vi "Avg_Example.vi"() -> ()   [LabVIEW 2019]
doc: "This example shows how to continously compute and show an averaged image.\nHere the camera class is operated in sequence mode and the required number of images also defines the number of images that will be averaged\nIt is a good starting point for writing own applications.\nBut it will not be fail save, i.e. doesnt react on errors, just handles them forward to the end\n\nUsage:\nSelect your required image count you want to average over before you start the program.\nOnce started, the camera class will be initialized and image record will start automatically.\nInside the acquisition loop the program will record the image sequence.\nThen it calculates the average image and shows it.\nBy using the ROI parameters you can crop the image to select certain regions\n\nBy clicking Quit Application the record will stop and will force an exit of the camera class"
uses:
  camera/Camera.lvclass
  <vilib>/picture/picture.llb/Draw 8-Bit Pixmap.vi
  <vilib>/picture/picture.llb/Draw True-Color Pixmap.vi
panel:
  out "colormap(U8)":u32[](array[numeric])
  out "Image(U16)":u16[][](graph)
  in  "Zoom [%]":i32(slide)=26 min=10 max=200 step=5 scale=10.0..200.0
  out "Image":picture
  out "rawImage":u16[][](array[numeric])
  in  "data_format":T1(ring)=enum."Mono16"
  out "Recorded Images":u32
  in  "Quit":bool
  in  "cropY1":u64=2 min=2 max=2048 step=1
  in  "cropX1":u64=2 min=2 max=2048 step=1
  in  "cropY0":u64=1 min=1 max=2047 step=1
  in  "cropX0":u64=1 min=1 max=2047 step=1
  out "Image Height":u64
  out "Image Width":u64
  in  "dwImgCount":u32=10 caption="Required Number of Images" max=4023
  out "Error":errorcluster {"code" format="%x"}
  # "This example shows how to continously compute and show an averaged image.\nHere the camera class is operated in sequence mode and the required number of images also defines the number of images that will be averaged\nIt is a good starting point for writing own applications.\nBut it will not be fail save, i.e. doesnt react on errors, just handles them forward to the end\n\nUsage:\nSelect your required image count you want to average over before you start the program.\nOnce started, the camera class will be initialized and image record will start automatically.\nInside the acquisition loop the program will record the image sequence.\nThen it calculates the average image and shows it.\nBy using the crop parameters you can crop the image to select certain regions\n\nBy clicking Quit Application the record will stop and will force an exit of the camera class"
  # "pco.labview"
  # "Camera Setup"
  # "Recording Control"
  # "Parameters for image readout"
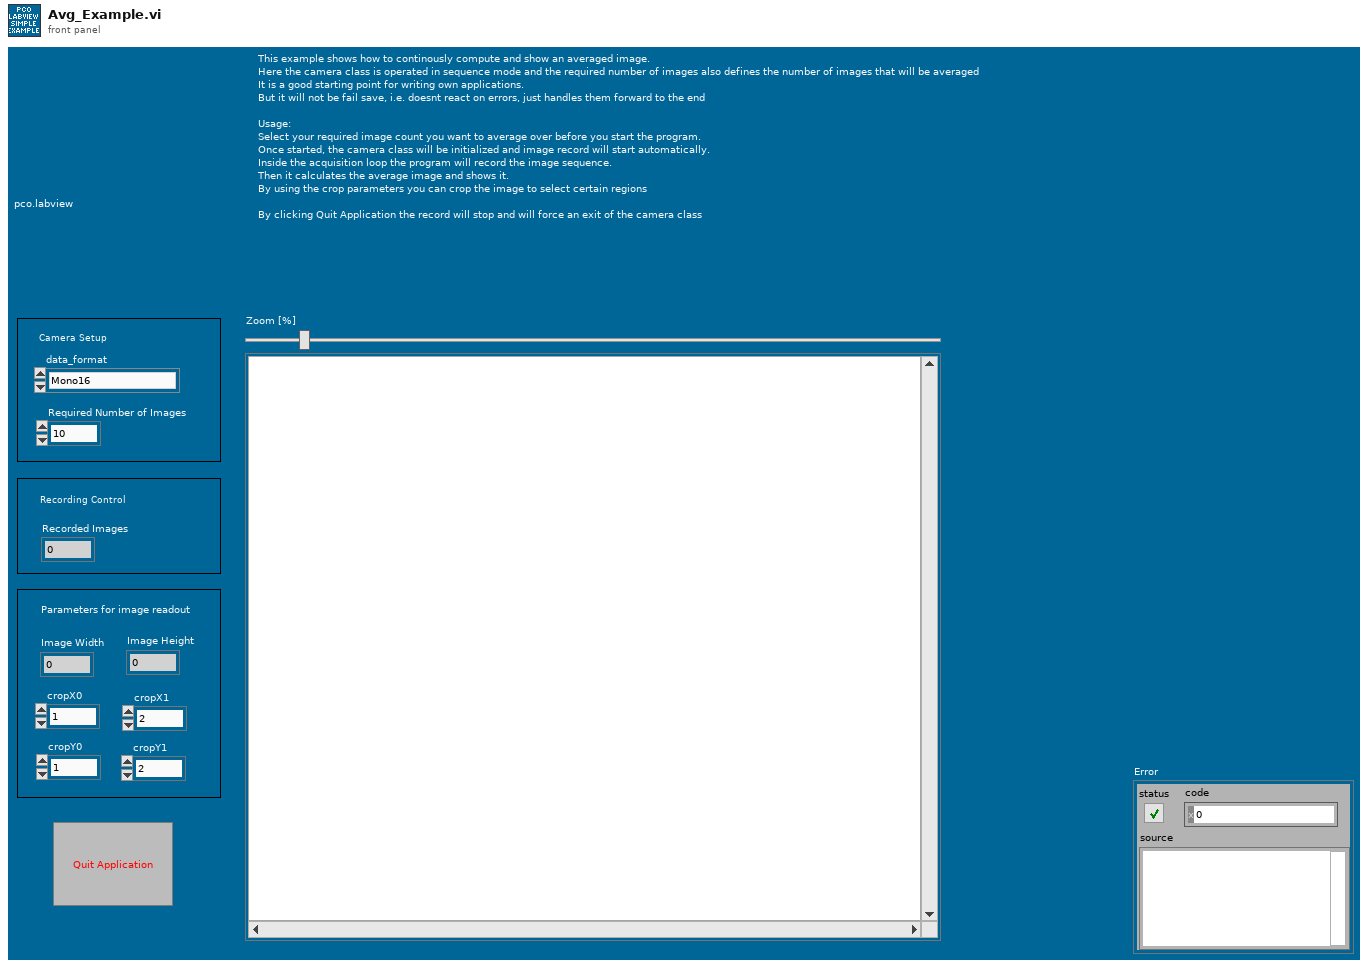
[diagram p1: front panel]
types:
  T1 = enum16{"Undefined", "Mono8", "Mono16", "BGRA8", "RGBA8", "BGRA16", "RGBA16", "CompressedMono8"}
  T2 = enum8{"Enabled", "Disabled", "Disabled and Grayed Out"}
  T3 = enum16{"sequence", "sequence non blocking", "ring buffer", "fifo", "tif", "multitif", "pcoraw", "b16", "dicom", "multidicom", "camram_ring", "camram_segment"}
  T4 = typedef "Camera.lvclass/binning.ctl" = cluster{"vert":u16, "horz":u16, "mode":u16}
  T5 = cluster{"exposure_time_s":dbl, "delay_time_s":dbl, "roi":cluster{"x0":u64, "y0":u64, "x1":u64, "y1":u64}, "timestamp_mode":u16, "pixelrate":u32, "conversion_factor":sgl, "trigger_mode":u16, "acquire_mode":u16, "acquire_sequence_number":u32, "metadata_mode":u16, "noisefilter_mode":u16, "pixel_format":u32, "binning":T4, "auto_exposure":cluster{"region":u16, "min_exposure_s":dbl, "max_exposure_s":dbl}}
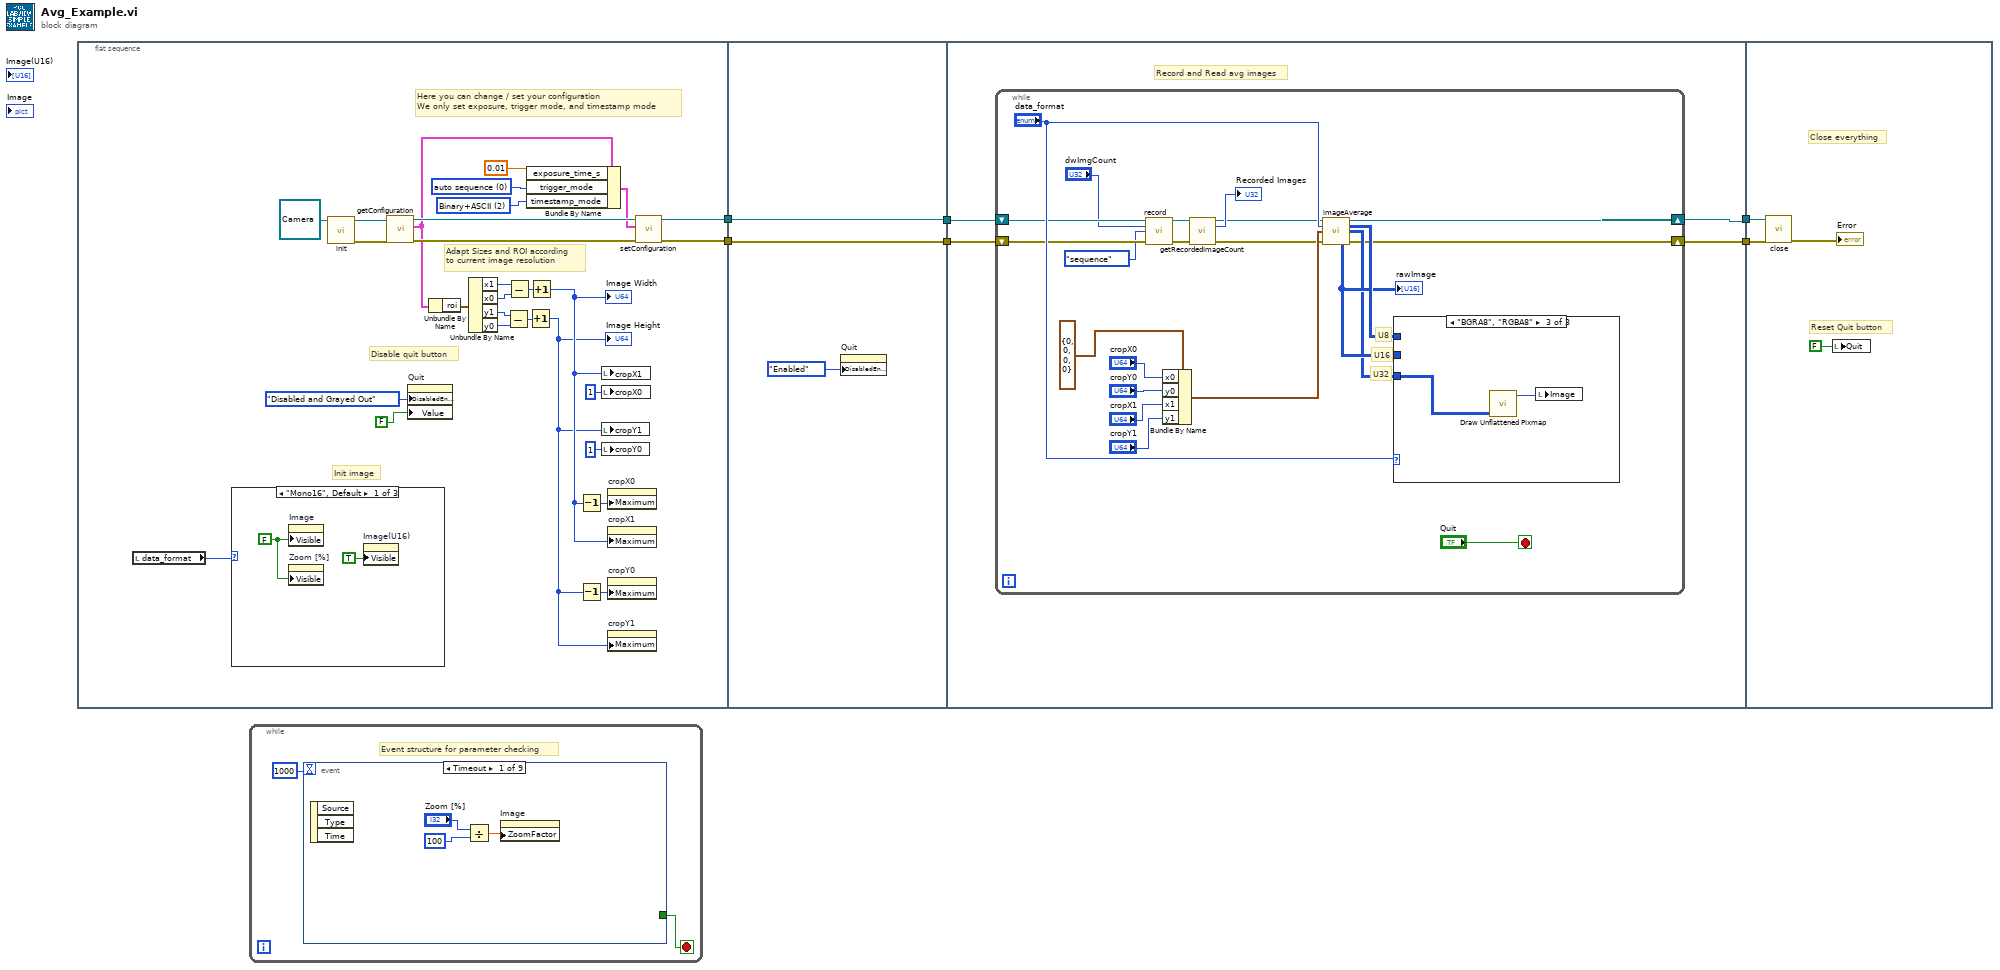
[diagram p0: block diagram]
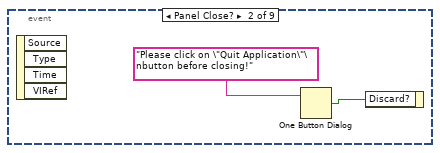
[diagram p2: hidden frame]
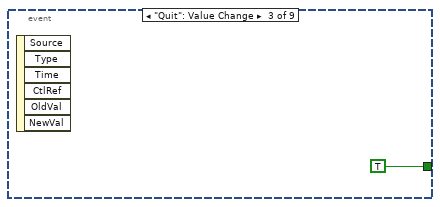
[diagram p3: hidden frame]
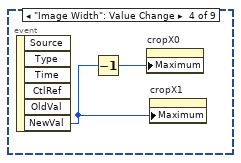
[diagram p4: hidden frame]
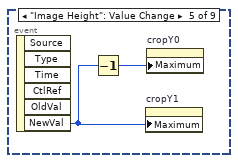
[diagram p5: hidden frame]
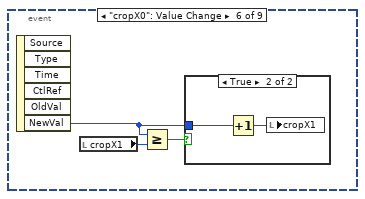
[diagram p6: hidden frame]
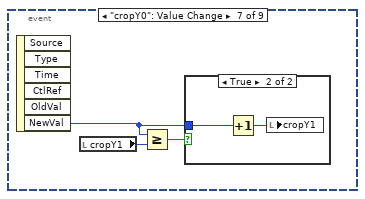
[diagram p8: hidden frame]
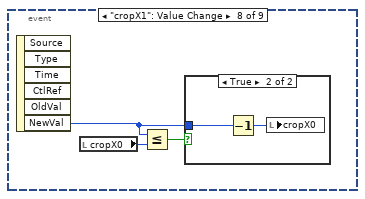
[diagram p10: hidden frame]
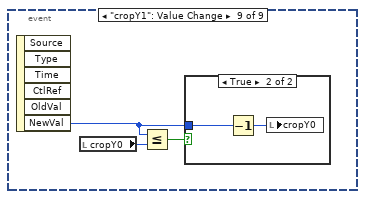
[diagram p12: hidden frame]
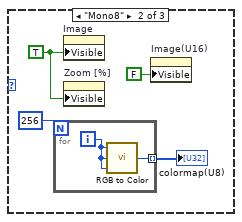
[diagram p14: hidden frame]
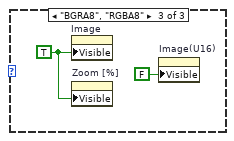
[diagram p15: hidden frame]
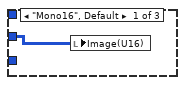
[diagram p16: hidden frame]
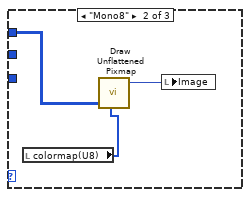
[diagram p17: hidden frame]
diagram:
  n1 = flat-sequence {
    tunnel: [w9] -> w6
    tunnel: [w8] -> w5
    tunnel: w6 -> [w46]
    tunnel: w5 -> [w45]
    tunnel: [w46] -> w4
    tunnel: [w45] -> w3
    tunnel: [w51] -> w2
    tunnel: [w50] -> w1
    tunnel: w3 -> [w49]
    tunnel: w4 -> [w48]
    tunnel: w2 -> [w81]
    tunnel: w1 -> [w80]
    frame #0 {
      w13 = u16 2 items=["OFF", "Binary", "Binary+ASCII", "ASCII"] ("TimestampMode")
      w31 = u16 0 items=["auto sequence"=0, "software trigger"=1, "external exposure start & software trigger"=2, "external exposure control"=3, "external synchronized"=4, "fast external exposure control"=5, "external CDS control"=6, "slow external exposure control"=7, "external synchronized HDSDI"=258] ("TriggerMode")
      # "Here you can change / set your configuration\nWe only set exposure, trigger mode, and timestamp mode"
      # "Init image"
      # "Adapt Sizes and ROI according\nto current image resolution"
      # "Disable quit button"
      n2 = local read "data_format"() -> (w10:T1)
      n3 = case shown="\"Mono16\", Default" w10 {
        frame "Mono16", Default {
          w35 = FALSE ("Visible")
          n4 = property on="Image" class="Pict"("Visible"=w35) -> ()  [unwired: 2 in, 2 out]
          n5 = property on="Zoom [%]" class="Slide (strict)"("Visible"=w35) -> ()  [unwired: 2 in, 2 out]
          n6 = property on="Image(U16)" class="IntGraph (strict)"("Visible"=TRUE) -> ()  [unwired: 2 in, 2 out]
        }
        frame "Mono8" {
          w39 = TRUE ("Visible")
          n7 = for {
            N: 256 -> [_]
            tunnel: [w41] -> w38 mode=indexing
            i -> [w42]
            n8 = call <vilib>:"RGB to Color.vi"("B"=w42, "G"=w42, "R"=w42) -> ("Color"=w41:u32)
          }
          "colormap(U8)" <- w38
          n9 = property on="Image" class="Pict"("Visible"=w39) -> ()  [unwired: 2 in, 2 out]
          n10 = property on="Zoom [%]" class="Slide (strict)"("Visible"=w39) -> ()  [unwired: 2 in, 2 out]
          n11 = property on="Image(U16)" class="IntGraph (strict)"("Visible"=FALSE) -> ()  [unwired: 2 in, 2 out]
        }
        frame "BGRA8", "RGBA8" {
          w43 = TRUE ("Visible")
          n12 = property on="Image" class="Pict"("Visible"=w43) -> ()  [unwired: 2 in, 2 out]
          n13 = property on="Zoom [%]" class="Slide (strict)"("Visible"=w43) -> ()  [unwired: 2 in, 2 out]
          n14 = property on="Image(U16)" class="IntGraph (strict)"("Visible"=FALSE) -> ()  [unwired: 2 in, 2 out]
        }
      }
      n15 = call-dynamic "init.vi"("Camera in"=refnum<class "Camera.lvclass"> refnum ("PCOCamera in")) -> ("Camera out"=w33:refnum<class "Camera.lvclass">, "error out"=w32:errorcluster)  [unwired: 8 in]
      n16 = call-dynamic "getConfiguration.vi"("error in (no error)"=w32, "Camera in"=w33) -> ("error out"=w29:errorcluster, "configuration"=w23:T5, "Camera out"=w30:refnum<class "Camera.lvclass">)  [unwired: 7 in]
      n17 = property on="Quit" class="Bool (strict)"("DisabledEnum"=T2."Disabled and Grayed Out" ("Disabled"), "Value"=FALSE ("Stop")) -> ()  [unwired: 2 in, 2 out]
      n18 = Unbundle By Name(w23) -> ("roi"=w22:cluster{"x0":u64, "y0":u64, "x1":u64, "y1":u64})
      n19 = Unbundle By Name(w22) -> ("x1"=w20:u64, "x0"=w21:u64, "y1"=w18:u64, "y0"=w19:u64)
      n20 = Subtract(x=w18, y=w19) -> (x-y=w16:u64)
      n21 = Subtract(x=w20, y=w21) -> (x-y=w17:u64)
      n22 = Bundle By Name(cluster=w23, "exposure_time_s"=0.01, "trigger_mode"=w31, "timestamp_mode"=w13) -> (w28:T5)
      n23 = Increment(x=w16) -> (x+1=w14:u64)
      "Image Height" <- w14
      n24 = Increment(x=w17) -> (x+1=w15:u64)
      "Image Width" <- w15
      n25 = Decrement(x=w15) -> (x-1=w25:u64)
      n26 = Decrement(x=w14) -> (x-1=w24:u64)
      n27 = local write "cropX1"(w15) -> ()
      n28 = local write "cropX0"(u64 1 ("roiY0")) -> ()
      n29 = local write "cropY1"(w14) -> ()
      n30 = local write "cropY0"(u64 1 ("roiY0")) -> ()
      n31 = property on="cropX0" class="DigNum (strict)"("Maximum"=w25) -> ()  [unwired: 2 in, 2 out]
      n32 = property on="cropX1" class="DigNum (strict)"("Maximum"=w15) -> ()  [unwired: 2 in, 2 out]
      n33 = property on="cropY0" class="DigNum (strict)"("Maximum"=w24) -> ()  [unwired: 2 in, 2 out]
      n34 = property on="cropY1" class="DigNum (strict)"("Maximum"=w14) -> ()  [unwired: 2 in, 2 out]
      n35 = call-dynamic "setConfiguration.vi"("error in (no error)"=w29, "configuration"=w28, "Camera in"=w30) -> ("error out"=w8:errorcluster, "Camera out"=w9:refnum<class "Camera.lvclass">)  [unwired: 7 in]
    }
    frame #1 {
      n36 = property on="Quit" class="Bool (strict)"("DisabledEnum"=T2."Enabled" ("Disabled")) -> ()  [unwired: 2 in, 2 out]
    }
    frame #2 {
      # "Record and Read avg images"
      n37 = while {
        shift-right: [w62] -> w51
        shift-left: w48 -> [w61]
        shift-right: [w53] -> w50
        shift-left: w49 -> [w60]
        stop <- "Quit" stop-if-true
        # "U32"
        # "U16"
        # "U8"
        n38 = call-dynamic "record.vi"("Camera in"=w61, "num_images"="dwImgCount", "record_mode"=T3."sequence", "error in (no error)"=w60) -> ("Camera out"=w59:refnum<class "Camera.lvclass">, "error out"=w58:errorcluster)  [unwired: 10 in]
        n39 = Bundle By Name(cluster=cluster{"x0":u64, "y0":u64, "x1":u64, "y1":u64} {"x0"=0, "y0"=0, "x1"=0, "y1"=0} ("roi"), "x0"="cropX0", "y0"="cropY0", "x1"="cropX1", "y1"="cropY1") -> (w69:cluster{"x0":u64, "y0":u64, "x1":u64, "y1":u64})
        n40 = call-dynamic "getRecordedImageCount.vi"("Camera in"=w59, "error in (no error)"=w58) -> ("Camera out"=w56:refnum<class "Camera.lvclass">, "recorded_image_count"=→"Recorded Images":u32, "error out"=w55:errorcluster)  [unwired: 11 in]
        n41 = call-dynamic "imageAverage.vi"("Camera in"=w56, "data_format"="data_format", "crop"=w69, "error in (no error)"=w55) -> ("Camera out"=w62:refnum<class "Camera.lvclass">, "image (U8)"=w67:u8[][], "image (U32)"=w65:u32[][], "raw_image (U16)"=w66:u16[][], "error out"=w53:errorcluster)  [unwired: 5 in, 2 out]
        "rawImage" <- w66
        n42 = case shown="\"BGRA8\", \"RGBA8\"" "data_format" {
          tunnel: w65 -> [_ _ w79]
          tunnel: w67 -> [_ w77 _]
          tunnel: w66 -> [w74 _ _]
          frame "Mono16", Default {
            n43 = local write "Image(U16)"(w74) -> ()
          }
          frame "Mono8" {
            n44 = local read "colormap(U8)"() -> (w75:u32[])
            n45 = call-poly <vilib>:"Draw Unflattened Pixmap.vi"("data"=w77, "color table"=w75) -> ("new picture"=w76:picture)  [unwired: 7 in]
            n46 = local write "Image"(w76) -> ()
          }
          frame "BGRA8", "RGBA8" {
            n47 = call-poly <vilib>:"Draw Unflattened Pixmap.vi"("data (RGB format)"=w79) -> ("new picture"=w78:picture)  [unwired: 8 in]
            n48 = local write "Image"(w78) -> ()
          }
        }
      }
    }
    frame #3 {
      # "Reset Quit button"
      # "Close everything"
      n49 = call-dynamic "close.vi"("error in (no error)"=w80, "Camera in"=w81) -> ("error out"=→"Error":errorcluster)  [unwired: 9 in]
      n50 = local write "Quit"(FALSE ("Stop")) -> ()
    }
  }
  n51 = while {
    stop <- w84 stop-if-true
    # "Event structure for parameter checking"
    n52 = event shown="[0] Timeout" {
      selector: _ -> [_ _ _ _ _ _ _ _ _]
      dyn-events: _ -> [_ _ _ _ _ _ _ _ _]
      timeout: 1000 -> [_ _ _ _ _ _ _ _ _]
      tunnel: [_ _ TRUE _ _ _ _ _ _] -> w84
      event Timeout {
        n53 = event-data() -> ()  [unwired: 1 in, 3 out]
        n54 = Divide(x="Zoom [%]", y=100 ("Zoom [%]")) -> (x/y=w87:dbl)
        n55 = property on="Image" class="Pict"("ZoomFactor"=w87) -> ()  [unwired: 2 in, 2 out]
      }
      event Panel Close? {
        n56 = event-data() -> ()  [unwired: 1 in, 4 out]
        n57 = One Button Dialog(message="Please click on \"Quit Application\"\nbutton before closing!") -> (true=w89:bool)  [unwired: 1 in]
        n58 = event-data("Discard?"=w89) -> ()  [unwired: 1 in, 1 out]
      }
      event "Quit": Value Change {
        n59 = event-data() -> ()  [unwired: 1 in, 6 out]
      }
      event "Image Width": Value Change {
        n60 = event-data() -> ("NewVal"=w92:u64)  [unwired: 1 in, 5 out]
        n61 = Decrement(x=w92) -> (x-1=w93:u64)
        n62 = property on="cropX0" class="DigNum (strict)"("Maximum"=w93) -> ()  [unwired: 2 in, 2 out]
        n63 = property on="cropX1" class="DigNum (strict)"("Maximum"=w92) -> ()  [unwired: 2 in, 2 out]
      }
      event "Image Height": Value Change {
        n64 = event-data() -> ("NewVal"=w94:u64)  [unwired: 1 in, 5 out]
        n65 = Decrement(x=w94) -> (x-1=w95:u64)
        n66 = property on="cropY1" class="DigNum (strict)"("Maximum"=w94) -> ()  [unwired: 2 in, 2 out]
        n67 = property on="cropY0" class="DigNum (strict)"("Maximum"=w95) -> ()  [unwired: 2 in, 2 out]
      }
      event "cropX0": Value Change {
        n68 = event-data() -> ("NewVal"=w96:u64)  [unwired: 1 in, 5 out]
        n69 = local read "cropX1"() -> (w98:u64)
        n70 = Greater Or Equal?(x=w96, y=w98) -> (x >= y?=w97:bool)
        n71 = case shown="True" w97 {
          tunnel: w96 -> [_ w100]
          frame False {
          }
          frame True {
            n72 = Increment(x=w100) -> (x+1=w99:u64)
            n73 = local write "cropX1"(w99) -> ()
          }
        }
      }
      event "cropY0": Value Change {
        n74 = event-data() -> ("NewVal"=w101:u64)  [unwired: 1 in, 5 out]
        n75 = local read "cropY1"() -> (w103:u64)
        n76 = Greater Or Equal?(x=w101, y=w103) -> (x >= y?=w102:bool)
        n77 = case shown="True" w102 {
          tunnel: w101 -> [_ w105]
          frame False {
          }
          frame True {
            n78 = Increment(x=w105) -> (x+1=w104:u64)
            n79 = local write "cropY1"(w104) -> ()
          }
        }
      }
      event "cropX1": Value Change {
        n80 = event-data() -> ("NewVal"=w106:u64)  [unwired: 1 in, 5 out]
        n81 = local read "cropX0"() -> (w108:u64)
        n82 = Less Or Equal?(x=w106, y=w108) -> (x <= y?=w107:bool)
        n83 = case shown="True" w107 {
          tunnel: w106 -> [_ w110]
          frame False {
          }
          frame True {
            n84 = Decrement(x=w110) -> (x-1=w109:u64)
            n85 = local write "cropX0"(w109) -> ()
          }
        }
      }
      event "cropY1": Value Change {
        n86 = event-data() -> ("NewVal"=w111:u64)  [unwired: 1 in, 5 out]
        n87 = local read "cropY0"() -> (w113:u64)
        n88 = Less Or Equal?(x=w111, y=w113) -> (x <= y?=w112:bool)
        n89 = case shown="True" w112 {
          tunnel: w111 -> [_ w115]
          frame False {
          }
          frame True {
            n90 = Decrement(x=w115) -> (x-1=w114:u64)
            n91 = local write "cropY0"(w114) -> ()
          }
        }
      }
    }
  }
